vi "reset Alarms.vi"(11 "devID":u32) -> (3 "function return":i32)   [LabVIEW 2014, in "libchaos-driver-powersupply-labview.lvlib"]
doc: "int resetAlarms(unsigned int devID);"
uses:
  libchaos-driver-powersupply-labview.lvlib
  chaos-i686-dynamic-release/lib/libchaos-driver-powersupply-labview.so
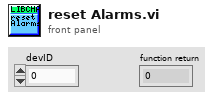
[diagram p1: front panel]
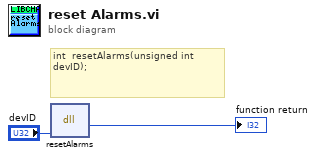
[diagram p0: block diagram]
diagram:
  # "int  resetAlarms(unsigned int devID);"
  n1 = dll-call lib="home/chaos/chaos_bundle/chaos-i686-dynamic-release/lib/libchaos-driver-powersupply-labview.*" fn="resetAlarms"("devID"="devID") -> (→"function return":i32)  [unwired: 4 in, 2 out]
